vi "CB Remote Sense Test.vi"(6 "Board Selector":T1, 7 "HMP4040 Channel Settings":T2={"CH1 Voltage"=24.0, "CH1 Current"=1.0, "CH1 Output"=TRUE, "CH2 Voltage"=24.0, "CH2 Current"=1.0, "CH2 Output"=TRUE, "CH3 Voltage"=24.0, "CH3 Current"=1.0, "CH3 Output"=TRUE, "CH4 Voltage"=24.0, "CH4 Current"=1.0, "CH4 Output"=TRUE, "Master Output"=TRUE} {"CH4 Current" format="%.3f"; "CH4 Voltage" format="%.3f"; "CH3 Current" format="%.3f"; "CH3 Voltage" format="%.3f"; "CH2 Current" format="%.3f"; "CH2 Voltage" format="%.3f"; "CH1 Current" format="%.3f"; "CH1 Voltage" format="%.3f"}, 8 "error in (no error)":errorcluster, 9 "VISA resource name":refnum<visa-resource-name>, 10 "Message IN":string) -> (0 "error out":errorcluster, 1 "Pass?":bool, 2 "Message OUT":string, 3 "Control Board OUT":refnum<visa-resource-name>)   [LabVIEW 2022 SP3]
uses:
  HMP4000 Communication/HMP4040_ChannelControl.ctl
  Serial Board Com/Board Select.ctl
panel:
  out "MSE Array":dbl[](array[numeric])
  out "Voltage Readings":dbl[][](array[numeric])
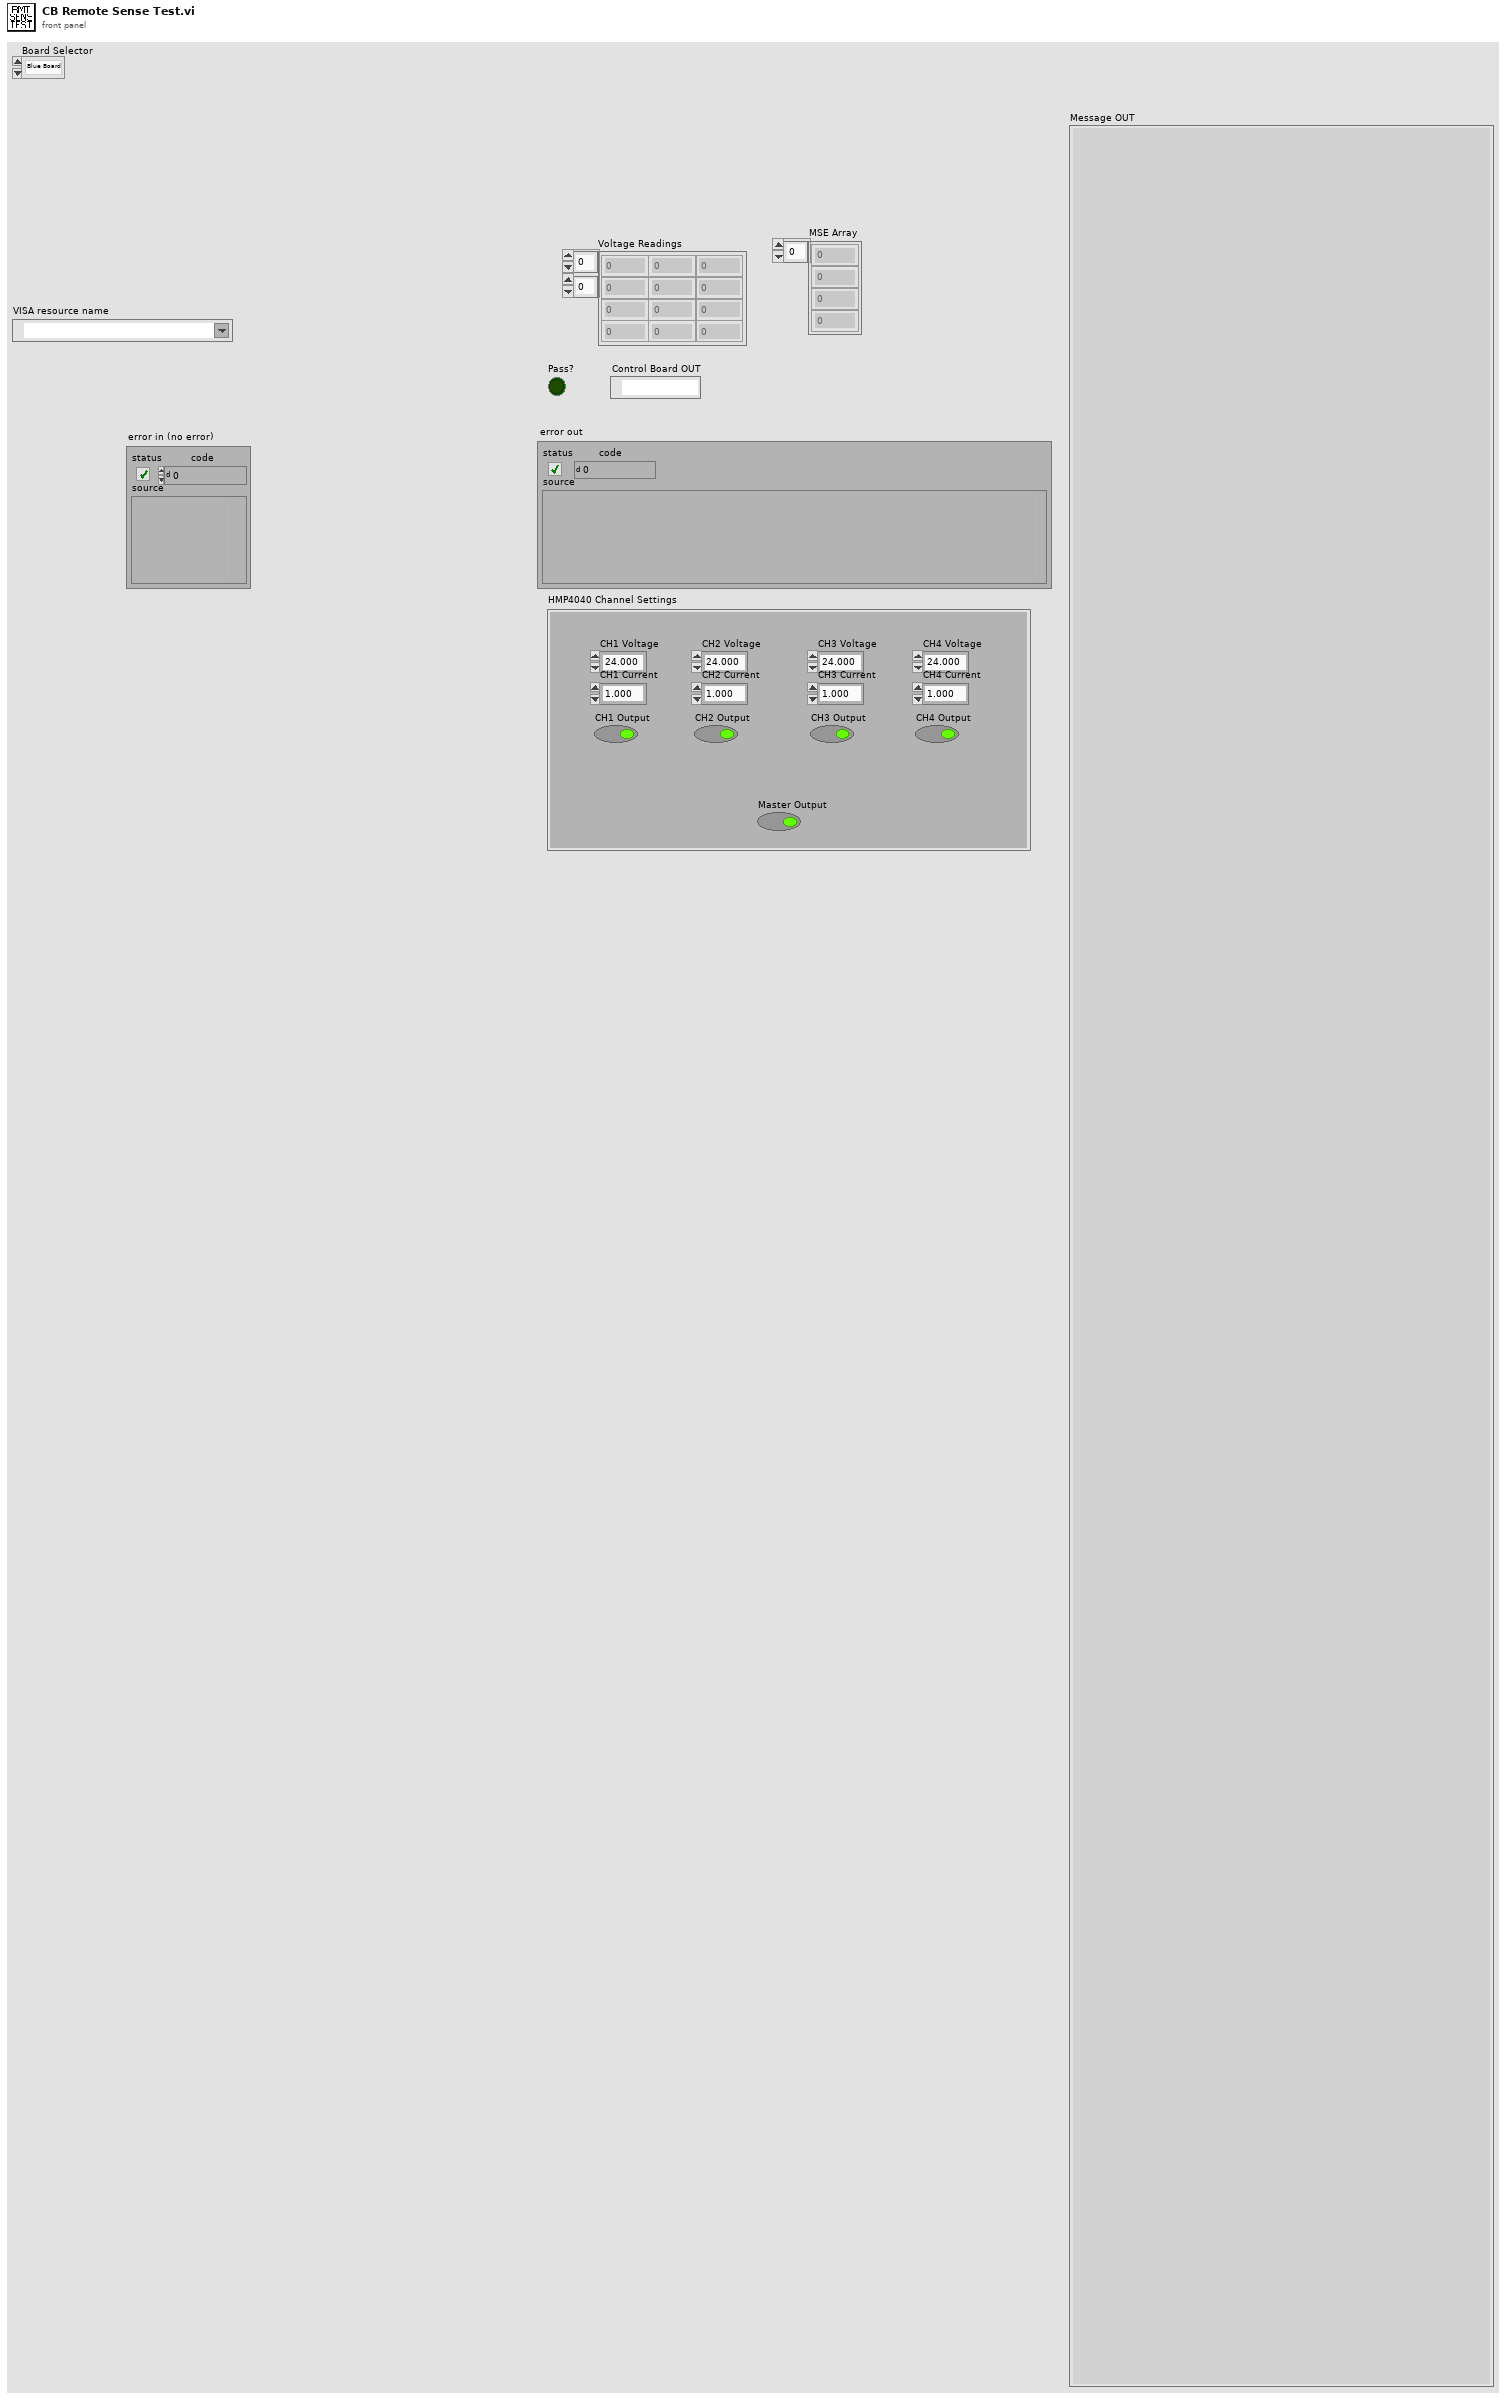
[diagram p1: front panel]
types:
  T1 = typedef "Board Select.ctl" = enum16{"Blue Board", "Green Board"}
  T2 = typedef "HMP4040_ChannelControl.ctl" = cluster{"CH1 Voltage":dbl, "CH1 Current":dbl, "CH1 Output":bool, "CH2 Voltage":dbl, "CH2 Current":dbl, "CH2 Output":bool, "CH3 Voltage":dbl, "CH3 Current":dbl, "CH3 Output":bool, "CH4 Voltage":dbl, "CH4 Current":dbl, "CH4 Output":bool, "Master Output":bool}
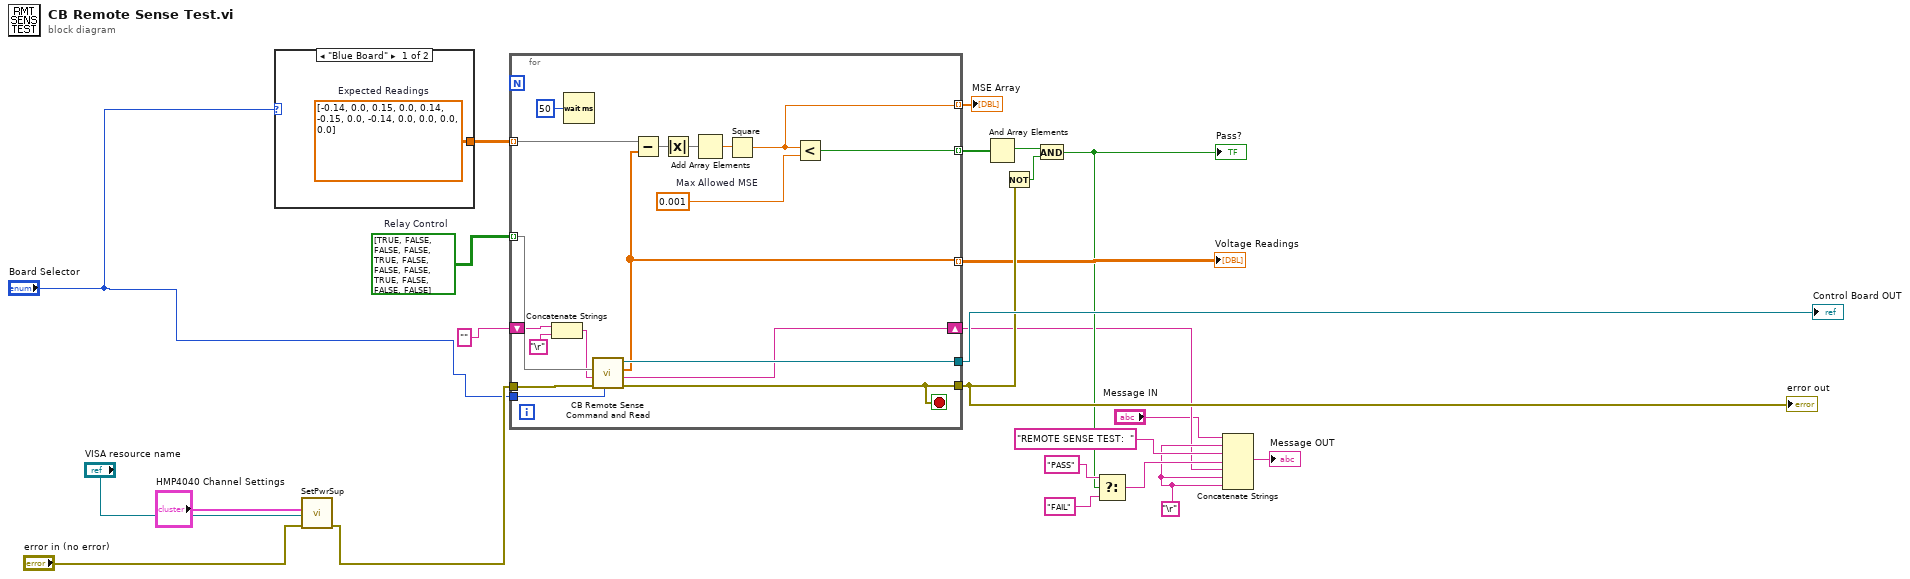
[diagram p0: block diagram]
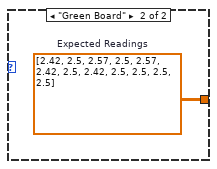
[diagram p2: hidden frame]
diagram:
  w10 = "\r"
  w21 = bool[][] [[TRUE, FALSE, FALSE], [FALSE, TRUE, FALSE], [FALSE, FALSE, TRUE], [FALSE, FALSE, FALSE]]  # Relay Control
  n1 = case shown="\"Blue Board\"" "Board Selector" {
    tunnel: [w25 w26] -> w23
    frame "Blue Board" {
      w25 = dbl[][] [[-0.14, 0.0, 0.15], [0.0, 0.14, -0.15], [0.0, -0.14, 0.0], [0.0, 0.0, 0.0]]  # Expected Readings
    }
    frame "Green Board" {
      w26 = dbl[][] [[2.42, 2.5, 2.57], [2.5, 2.57, 2.42], [2.5, 2.42, 2.5], [2.5, 2.5, 2.5]]  # Expected Readings
    }
  }
  n2 = call "SetPwrSup.vi"("error in (no error)"="error in (no error)", "HMP4040 Channel Settings"="HMP4040 Channel Settings", "HMP4040 IN"="VISA resource name") -> ("error out"=w4:errorcluster)  [unwired: 7 in, 1 out]
  n3 = for {
    tunnel: [w42] -> w18
    tunnel: [w44] -> w24
    tunnel: w4 -> [w43]
    tunnel: w23 -> [w39] mode=indexing
    tunnel: [w36] -> w22 mode=indexing
    tunnel: w21 -> [w35] mode=indexing
    tunnel: [w34] -> w17 mode=indexing
    tunnel: [w33] -> w16 mode=indexing
    shift-right: [w32] -> w8
    shift-left: "" -> [w31]
    tunnel: "Board Selector" -> [w28]
    stop <- w42 stop-if-true
    w37 = 0.001  # Max Allowed MSE
    n4 = Concatenate Strings(w31, "\r") -> (w30:string)
    n5 = Wait (ms)(milliseconds to wait=u32 50) -> ()  [unwired: 1 out]
    n6 = call "CB Remote Sense Command and Read.vi"("Board Selector"=w28, "error in (no error)"=w43, "Message IN"=w30, "Relay Control"=w35) -> ("error out"=w42:errorcluster, "Message OUT"=w32:string, "Voltage Array"=w34:dbl[], "Control Board OUT"=w44:refnum<visa-resource-name>)  [unwired: 4 in]
    n7 = Subtract(x=w39, y=w34) -> (x-y=w41:dbl[])
    n8 = Absolute Value(x=w41) -> (abs(x)=w40:dbl[])
    n9 = Add Array Elements(numeric array=w40) -> (sum=w38:dbl)
    n10 = Square(x=w38) -> (x^2=w33:dbl)
    n11 = Less?(x=w33, y=w37) -> (x < y?=w36:bool)
  }
  "error out" <- w18
  "Voltage Readings" <- w17
  "MSE Array" <- w16
  "Control Board OUT" <- w24
  n12 = And Array Elements(Boolean array=w22) -> (logical AND=w20:bool)
  n13 = Not(x=w18) -> (.not. x?=w19:bool)
  n14 = And(x=w20, y=w19) -> (x .and. y?=w9:bool)
  "Pass?" <- w9
  n15 = Select(t="PASS", s=w9, f="FAIL") -> (s? t:f=w14:string)
  n16 = Concatenate Strings("Message IN", w10, "REMOTE SENSE TEST:  ", w14, w8, w10, w10) -> (→"Message OUT":string)
